vi "stateMachine_dualVStim_beta2.vi"() -> ()   [LabVIEW 2014]
uses:
  daq_channel_read_parameter.ctl
  <vilib>/Platform/TimedLoop/XDataNode/timing_clust.ctl
  <vilib>/Platform/TimedLoop/XDataNode/nitl_modes.ctl
  <vilib>/Platform/TimedLoop/XDataNode/wakeup.ctl
  <vilib>/dex/Stream Element Allocation Mode.ctl
  states_def.ctl
  UDP_Para_def.ctl
  <vilib>/DAQmx/write.llb/DAQmx Write (Digital 1D Bool NChan 1Samp 1Line).vi
  <vilib>/platform/TimedLoop/XDataNode/XDataNode.xnode
  <vilib>/Platform/TimedLoop/XDataNode/XDNodeRunTimeDep.lvlib
  <resource>/objmgr/ni.dex.rc
panel:
  out "rightcounter":i32
  out "leftcounter":i32
  out "beh type":string
  out "vs type":string
  out "Tab Control":enum32{"State Machine"}(tab)
  in  "No VS":bool
  in  "vsFilterPeriod_uS":i32=500 format="%#1.6f"
  in  "lickThreshold_V":fxp<+/-,16,5> format="%#.4g"
  in  "vsThreshold_V":fxp<+/-,16,5> format="%#.4g"
  in  "audioThreshold_V":fxp<+/-,16,5> format="%#.4g"
  in  "audioFilterPeriod_uS":i32=50000 format="%#1.6f"
  in  "audioOffState_V":fxp<+/-,16,5> format="%#.4g"
  out "rtFIFOsize":u32=50
  out "rtFIFOtimeout":u32
  out "rtFIFOdataPool":u32=50
  out "stateMachineCycle_uS":i64=500
  out "(Actual)":i64
  in  "delay_uS":u32
  out "IP_RT":string="192.168.137.2"
  in  "port_broadcast":u16=9091
  out "IP_host":string="192.168.137.1"
  out "port_host":u16=9090
  in  "Tab Control 2":enum32{"Data Transfer"}(tab)
  out "stream counter":u32
  out "Is Connected":bool
  out "Available Elements for Writing":i32
  out "stream writer buffer size":i32=500
  in  "rewardPeriod_uS":u32
  in  "waterOn_uS":u32
  in  "timeout_uS":u32=5000000
  in  "shockOn_uS":u32
  in  "Stop state":bool
  out "Initial data received":bool
  out "Tab Control 3":enum32{"Current status"}(tab)
  in  "toneReward":bool
  out "ABORT":bool
  out "trialStart":bool
  out "trialDone":bool
  out "Busy":bool
  out "stateLatched":bool
  out "curKey":u32=1
  out "curState":u32
  out "rtFIFOdataDim":i32
  in  "actuatorOn":bool
  in  "manualWaterRight":bool
  in  "manualWaterLeft":bool
  in  "lickReward":bool
  in  "allowPunish":bool
  in  "forceLRswitch":bool
  in  "allowCorrection":bool
  in  "allowAutoWater":bool
  out "error out":errorcluster
  in  "trialKey":i32[](array[numeric])
  in  "rwdrefPeriod_uS":u32
  out "FlagWaterLeft":bool
  in  "chanellParaCluster":T1={"audioOffState_V"=0.0, "audioFilterPeriod_uS"=50000, "audioThreshold_V"=0.0, "vsThreshold_V"=0.0, "vsFilterPeriod_uS"=0, "lickThreshold_V"=0.0} {"vsFilterPeriod_uS" format="%#1.6f"; "audioFilterPeriod_uS" format="%#1.6f"}
  out "leftWaterOnFlag":bool
  out "rightWaterOnFlag":bool
  out "contNoReward":i32
  out "rewardStatus":bool
  in  "timeVS_uS":u32=2000000
  in  "timeTravel_uS":i32=400000
  out "skipRewFlag":bool
types:
  T1 = typedef "daq_channel_read_parameter.ctl" = cluster{"audioOffState_V":fxp<+/-,16,5>, "audioFilterPeriod_uS":i32, "audioThreshold_V":fxp<+/-,16,5>, "vsThreshold_V":fxp<+/-,16,5>, "vsFilterPeriod_uS":i32, "lickThreshold_V":fxp<+/-,16,5>}
  T2 = typedef "XDNodeRunTimeDep.lvlib/timing_clust.ctl" = cluster{"Expected End [f-1]":u64, "Actual End [f-1]":u64, "Finished Late? [f-1]":bool, "Expected End [i-1]":u64, "Actual End [i-1]":u64, "Finished Late? [i-1]":bool, "Expected Start [i]":u64, "Actual Start [i]":u64, "Expected Start [f]":u64, "Actual Start [f]":u64, "Source Name":string, "Structure Name":string, "Period":i64, "Deadline":i64, "Offset":i64, "Start":i64, "Priority":i32, "Timeout":i32, "Mode":T3, "Wakeup Reason":T4, "Error":errorcluster, "Source Type":string, "Secondary Source Type":string, "Global End Time":u64, "Global Start Time":u64, "Frame Duration":u64, "Iteration Duration":u64, "Assigned CPU":i32, "I/O Scan Engine Mode":u32}
  T3 = typedef "XDNodeRunTimeDep.lvlib/nitl_modes.ctl" = enum32{"No Change", "Process missed periods, maintain original phase", "Discard missed periods, maintain original phase", "Process missed periods, ignore original phase", "Discard missed periods, ignore original phase"}
  T4 = typedef "XDNodeRunTimeDep.lvlib/wakeup.ctl" = enum32{"Normal", "Aborted", "Asynchronous wakeup", "Timing source error", "Timed loop error", "Timeout"}
  T5 = typedef "states_def.ctl" = enum16{"idle", "vs before", "vs", "vs after", "delay", "tone before", "tone", "tone after", "cycle end", "reward", "reward refractory", "punish", "punish refractory", "timeout", "exit", "manualwater"}
  T6 = typedef "Stream Element Allocation Mode.ctl" = u32
  T7 = typedef "UDP_Para_def.ctl" = enum16{"no", "start", "stop", "dly", "rwp", "rwf", "wdr", "shd", "tod", "lkr", "tlr", "alp", "msh", "mwl", "mwr", "alc", "lth", "vth", "ath", "aof", "afp", "vfp"}
  T8 = cluster{"leftLick":bool, "rightLick":bool, "visualStimuli2":bool, "tone":bool, "visualStimuli1":bool}
  T9 = cluster{"leftLick":dbl, "rightLick":dbl, "visualStimuli2":dbl, "tone":dbl, "visualStimuli1":dbl}
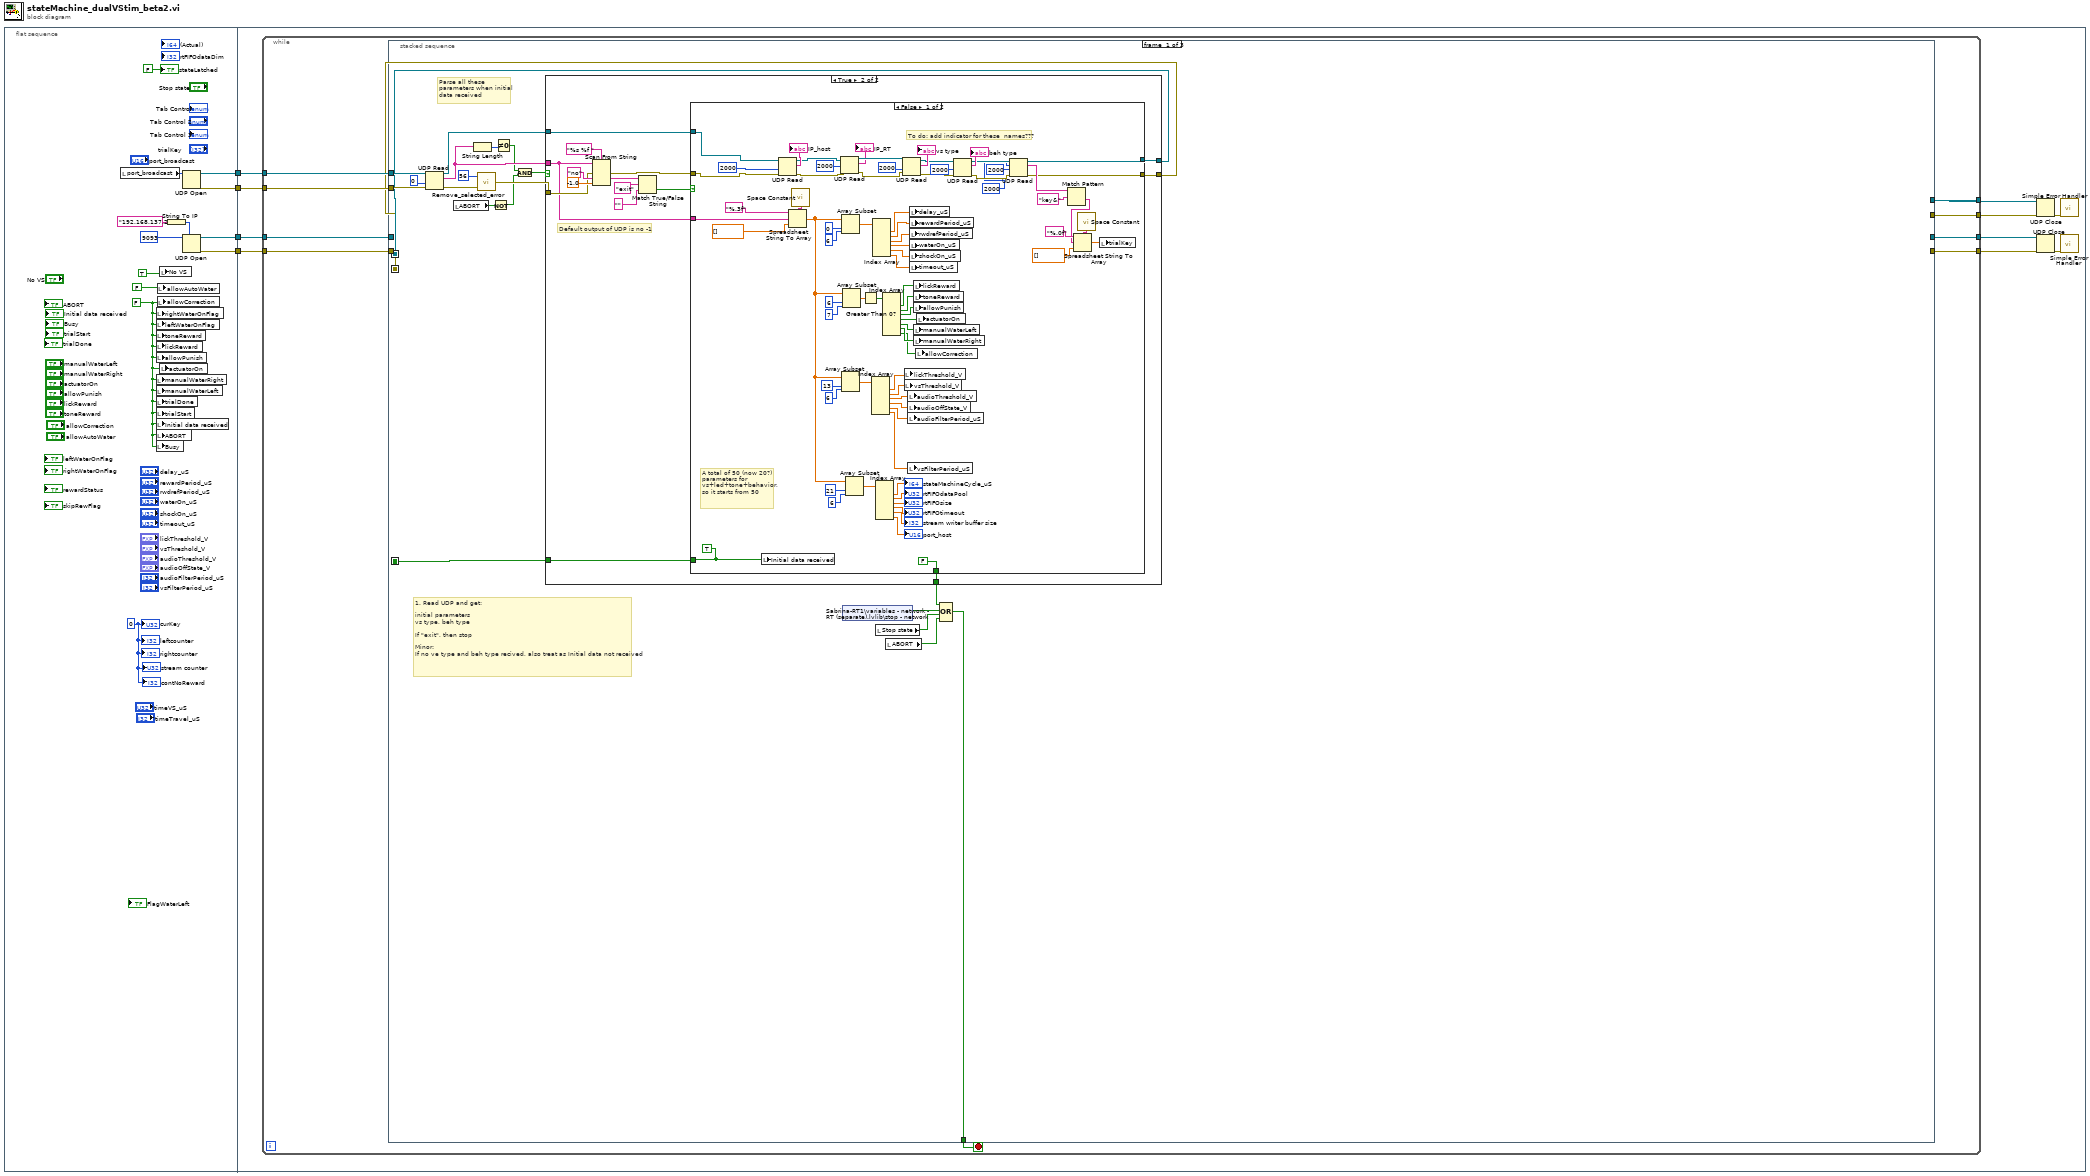
[diagram p0: block diagram]
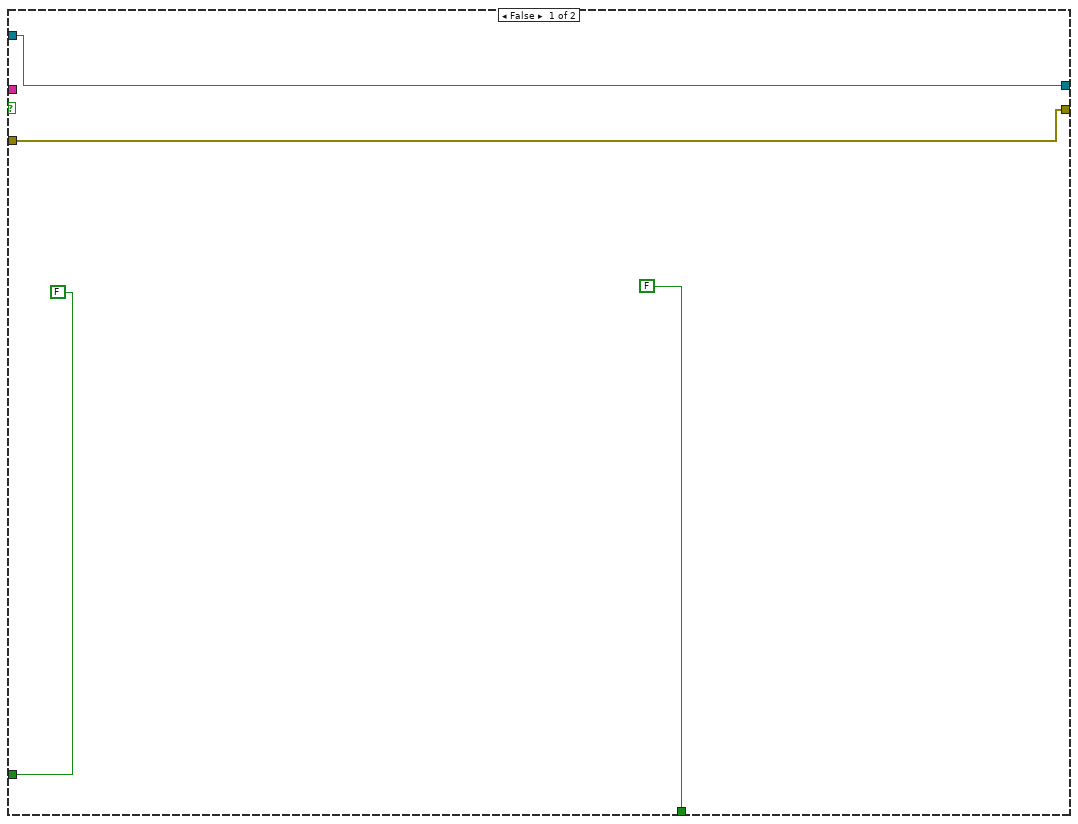
[diagram p2: hidden frame]
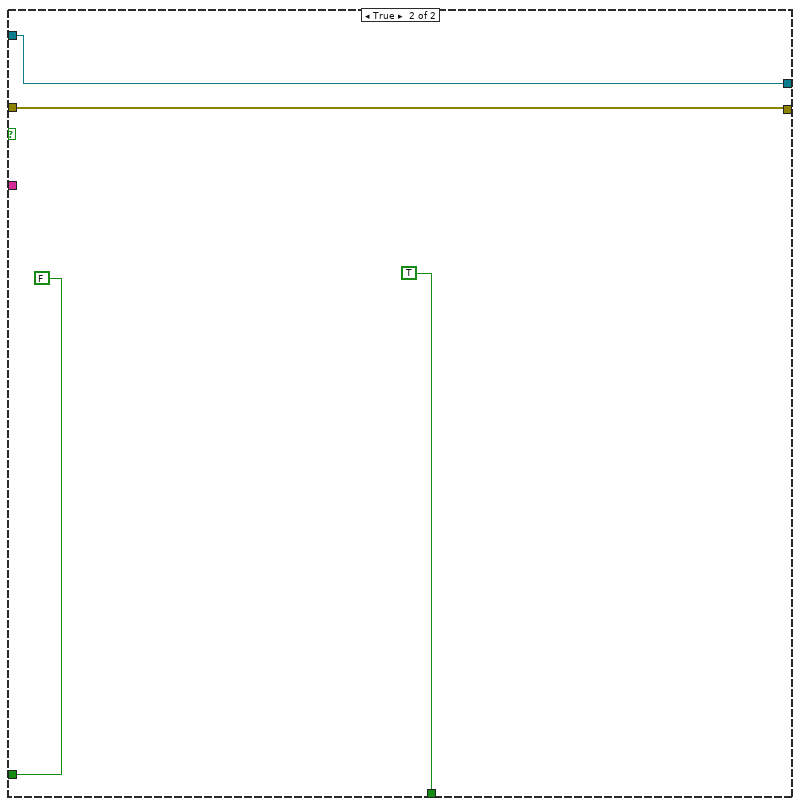
[diagram p3: hidden frame]
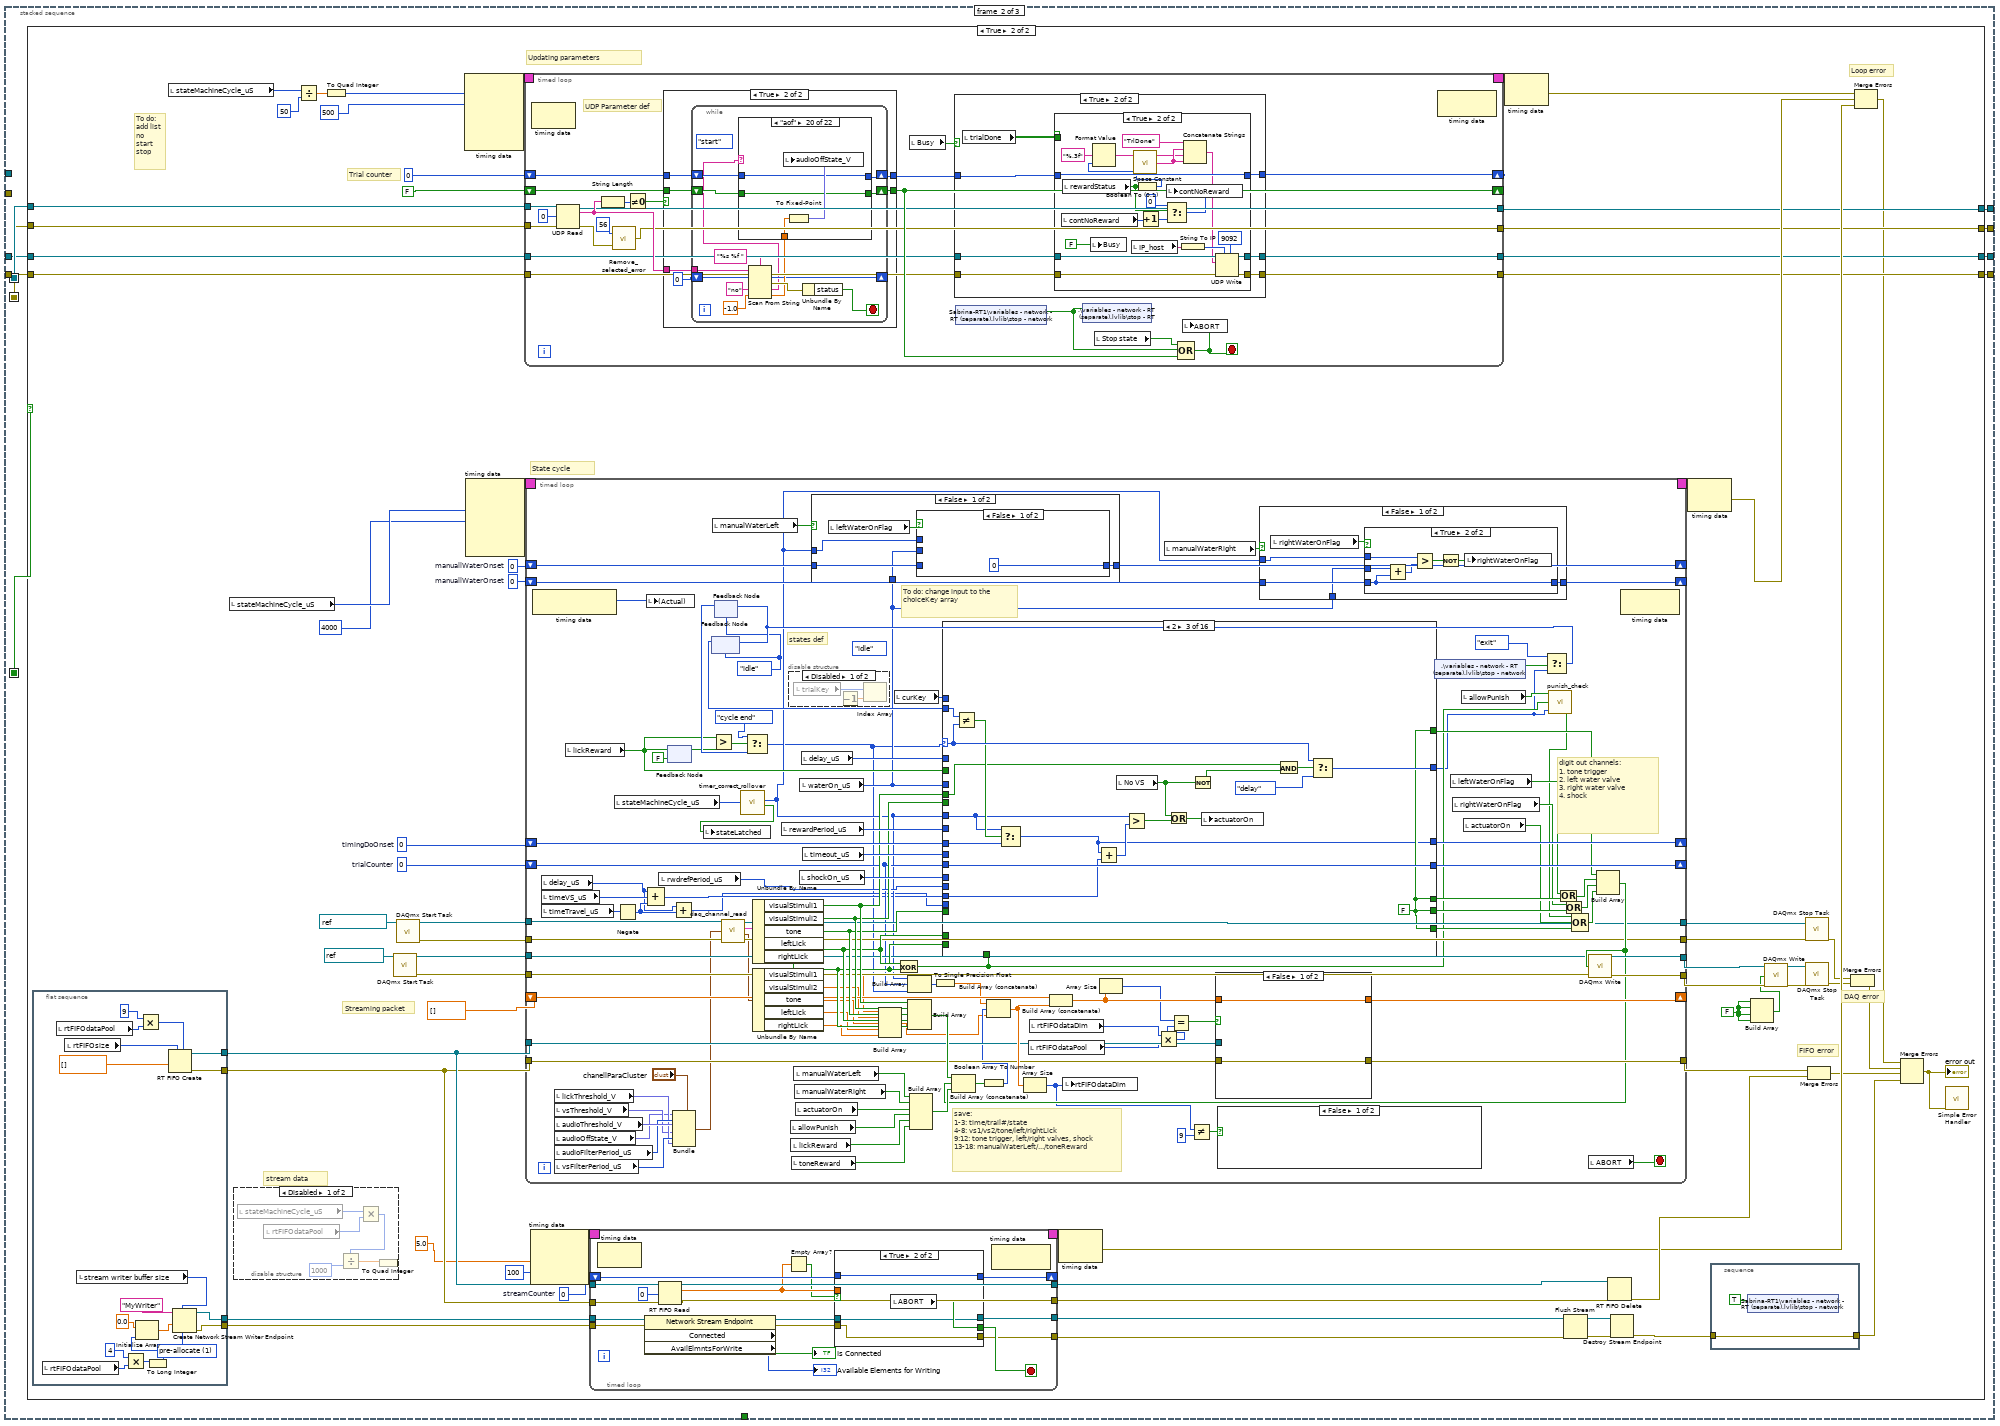
[diagram p4: hidden frame]
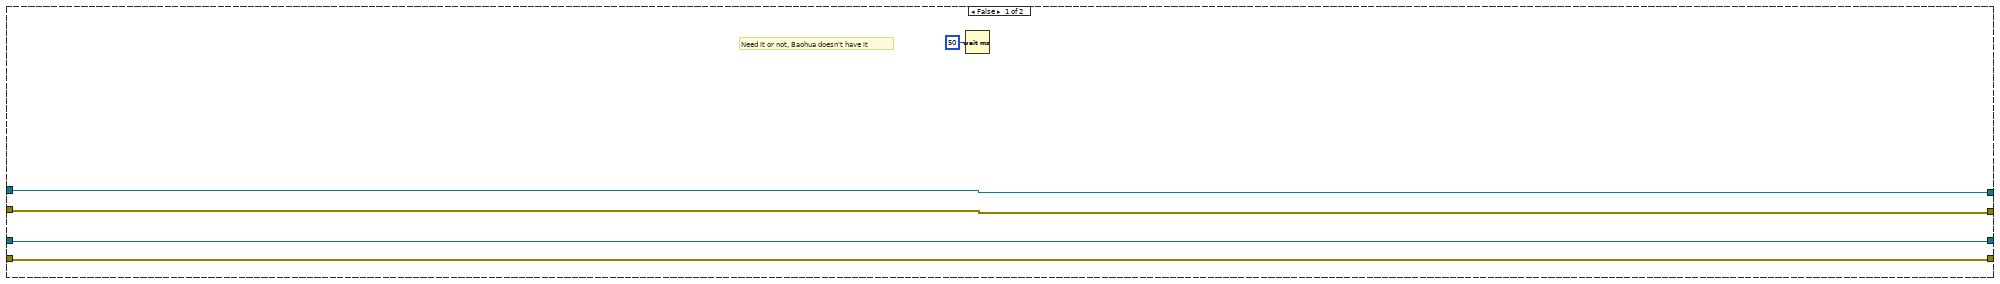
[diagram p5: hidden frame]
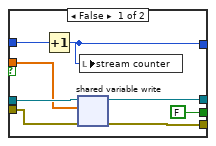
[diagram p7: hidden frame]
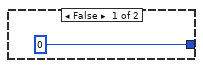
[diagram p9: hidden frame]
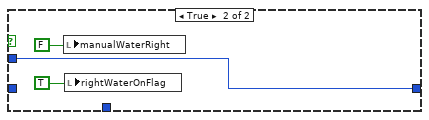
[diagram p10: hidden frame]
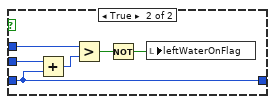
[diagram p11: hidden frame]
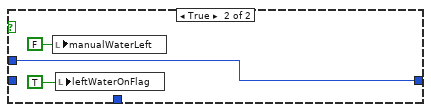
[diagram p12: hidden frame]
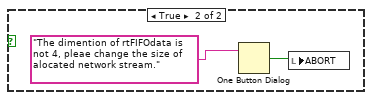
[diagram p13: hidden frame]
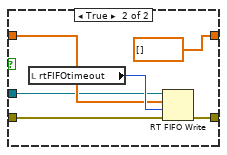
[diagram p14: hidden frame]
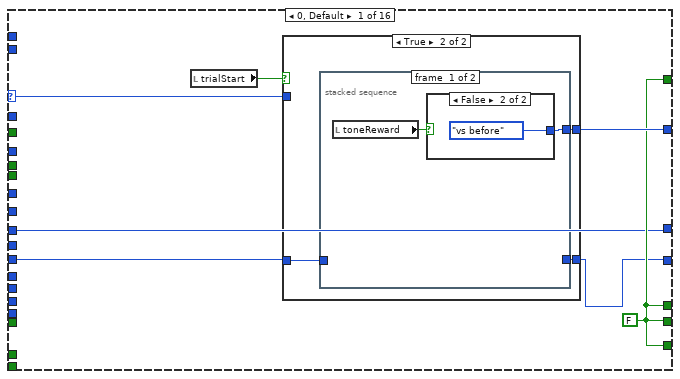
[diagram p15: hidden frame]
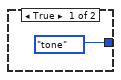
[diagram p17: hidden frame]
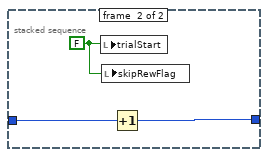
[diagram p18: hidden frame]
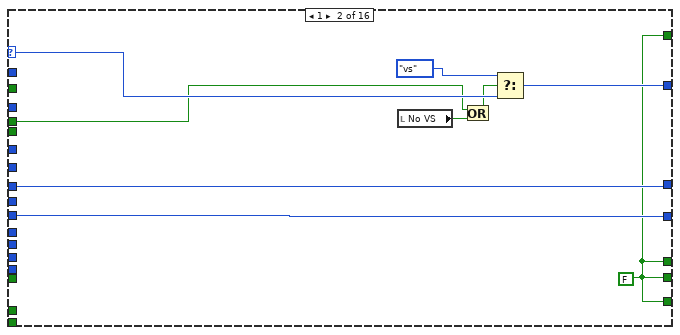
[diagram p19: hidden frame]
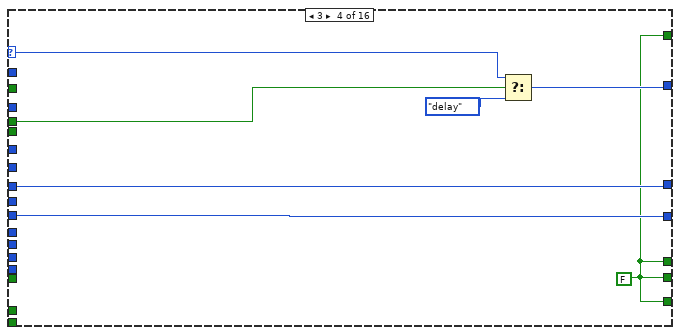
[diagram p20: hidden frame]
diagram:
  n1 = flat-sequence {
    tunnel: [w17] -> w4
    tunnel: [w16] -> w3
    tunnel: [w12] -> w2
    tunnel: [w11] -> w1
    tunnel: w4 -> [w27]
    tunnel: w3 -> [w26]
    tunnel: w2 -> [w22]
    tunnel: w1 -> [w21]
    frame #0 {
      w8 = FALSE
      w7 = 0
      n2 = local read "port_broadcast"() -> (w15:u16)
      n3 = local write "rightWaterOnFlag"(w8) -> ()
      n4 = local write "leftWaterOnFlag"(w8) -> ()
      n5 = local write "toneReward"(w8) -> ()
      n6 = local write "lickReward"(w8) -> ()
      n7 = local write "allowPunish"(w8) -> ()
      n8 = local write "manualWaterRight"(w8) -> ()
      n9 = local write "manualWaterLeft"(w8) -> ()
      n10 = local write "trialDone"(w8) -> ()
      n11 = local write "trialStart"(w8) -> ()
      n12 = local write "Initial data received"(w8) -> ()
      n13 = local write "ABORT"(w8) -> ()
      n14 = local write "Busy"(w8) -> ()
      n15 = local write "allowAutoWater"(FALSE) -> ()
      n16 = local write "allowCorrection"(w8) -> ()
      n17 = local write "No VS"(TRUE) -> ()
      n18 = local write "actuatorOn"(w8) -> ()
      n19 = String To IP(1:"192.168.137.2") -> (0:w9:u32)
      n20 = UDP Open(7:w9, 11:u16 9093) -> (port=w12:refnum<k16>, 0:w11:errorcluster)  [unwired: 3 in, 1 out]
      n21 = UDP Open(11:w15) -> (port=w17:refnum<k16>, 0:w16:errorcluster)  [unwired: 4 in, 1 out]
      "stateLatched" <- FALSE
      "curKey" <- w7
      "leftcounter" <- w7
      "rightcounter" <- w7
      "stream counter" <- w7
      "contNoReward" <- w7
    }
    frame #1 {
      n22 = while {
        tunnel: w27 -> [w36]
        tunnel: w26 -> [w35]
        tunnel: [w33] -> w24
        tunnel: [w32] -> w23
        tunnel: w22 -> [w31]
        tunnel: w21 -> [w30]
        tunnel: [w29] -> w20
        tunnel: [w28] -> w19
        stop <- w34 stop-if-true
        n23 = stacked-sequence {
          seq-local: [w46 _ _] -> [_ w163 _]
          seq-local: [w38 _ _] -> [_ w160 _]
          seq-local: [w37 _ _] -> [_ w159 _]
          tunnel: w36 -> [w57 _ _]
          tunnel: w35 -> [w56 _ _]
          tunnel: [w47 _ _] -> w34
          tunnel: [_ w162 _] -> w33
          tunnel: [_ w161 _] -> w32
          tunnel: w31 -> [_ w158 _]
          tunnel: w30 -> [_ w155 _]
          tunnel: [_ w157 _] -> w29
          tunnel: [_ w156 _] -> w28
          frame #0 {
            # "Parse all these \nparameters when initial\ndata received"
            # "1. Read UDP and get:\n\ninitial parameters\nvs type, beh type\n\nIf \"exit\", then stop\n\nMinor:\nIf no ve type and beh type recived, also treat as Initial data not received"
            n24 = UDP Read(connection ID=w57, timeout ms (25000)=0, 8:w56) -> (data out=w54:string, error out=w44:errorcluster, 3:w55:refnum<k16>)  [unwired: 1 in, 2 out]
            n25 = local read "ABORT"() -> (w42:bool)
            n26 = String Length(string=w54) -> (length=w53:i32)
            n27 = call "Remove_selected_error.vi"("error in (no error)"=w44, "errorCode"=56 ("timeout ms (25000)")) -> ("error out"=w45:errorcluster)
            n28 = Not(x=w42) -> (.not. x?=w39:bool)
            n29 = Not Equal To 0?(x=w53) -> (x != 0?=w40:bool)
            n30 = And(x=w40, y=w39) -> (x .and. y?=w41:bool)
            n31 = case shown="True" w41 {
              tunnel: w54 -> [_ w66]
              tunnel: w55 -> [w59 w67]
              tunnel: w45 -> [w58 w74]
              tunnel: [FALSE w65] -> w51
              tunnel: [FALSE w64] -> w46
              tunnel: [w59 w63] -> w38
              tunnel: [w58 w62] -> w37
              frame False {
              }
              frame True {
                # "Default output of UDP is no -1"
                n32 = Scan From String(format string="%s %f ", input string=w66, error in=w74, default 1="no" ("default value 1"), default 2=sgl -1.0 ("default value 1")) -> (error out=w68:errorcluster, output 1=w73:string)  [unwired: 2 in, 2 out]
                n33 = Match True/False String(2:"" ("false string"), 3:"exit" ("true string"), 4:w73) -> (0:w69:bool)  [unwired: 1 out]
                n34 = case shown="False" w69 {
                  tunnel: w68 -> [w112 w152]
                  tunnel: w67 -> [w113 w151]
                  tunnel: w66 -> [w144 _]
                  tunnel: [FALSE TRUE] -> w65
                  tunnel: [w142 FALSE] -> w64
                  tunnel: [w79 w151] -> w63
                  tunnel: [w78 w152] -> w62
                  frame False {
                    w142 = TRUE
                    # "A total of 50 (now 20?) parameters for vs+led+tone+behavior, so it starts from 50"
                    # "To do: add indicator for these  names???"
                    n35 = local write "Initial data received"(w142) -> ()
                    n36 = UDP Read(connection ID=w113, timeout ms (25000)=2000, 8:w112) -> (data out=→"IP_host":string, error out=w111:errorcluster, 3:w109:refnum<k16>)  [unwired: 1 in, 2 out]
                    n37 = call <vilib>:"Space Constant.vi"() -> ("String"=w149:string)
                    n38 = Spreadsheet String To Array(delimiter (Tab)=w149, format string="%.3f", spreadsheet string=w144, array type (2D Dbl)=sgl[] []) -> (array=w120:sgl[])
                    n39 = UDP Read(connection ID=w109, timeout ms (25000)=2000, 8:w111) -> (data out=→"IP_RT":string, error out=w110:errorcluster, 3:w108:refnum<k16>)  [unwired: 1 in, 2 out]
                    n40 = Array Subset(array=w120, index=0 ("timeout ms (25000)"), length=6 ("timeout ms (25000)")) -> (w138:sgl[])
                    n41 = Array Subset(array=w120, index=13 ("timeout ms (25000)"), length=6 ("timeout ms (25000)")) -> (w134:sgl[])
                    n42 = Array Subset(array=w120, index=6 ("timeout ms (25000)"), length=7 ("timeout ms (25000)")) -> (w131:sgl[])
                    n43 = Array Subset(array=w120, index=21 ("timeout ms (25000)"), length=6 ("timeout ms (25000)")) -> (w121:sgl[])
                    n44 = Greater Than 0?(x=w131) -> (x > 0?=w130:bool[])
                    n45 = Index Array(array=w134) -> (element #1=w96:sgl, element #2=w95:sgl, element #3=w94:sgl, element #4=w93:sgl, element #5=w92:sgl, element #6=w91:sgl)  [unwired: 6 in]
                    n46 = Index Array(array=w138) -> (element #1=w102:sgl, element #2=w101:sgl, element #3=w100:sgl, element #4=w99:sgl, element #5=w98:sgl, element #6=w97:sgl)  [unwired: 6 in]
                    n47 = Index Array(array=w121) -> (element #1=→"stateMachineCycle_uS":sgl, element #2=→"rtFIFOdataPool":sgl, element #3=→"rtFIFOsize":sgl, element #4=→"rtFIFOtimeout":sgl, element #5=→"stream writer buffer size":sgl, element #6=→"port_host":sgl)  [unwired: 6 in]
                    n48 = Index Array(array=w130) -> (element #1=w129:bool, element #2=w128:bool, element #3=w127:bool, element #4=w126:bool, element #5=w125:bool, element #6=w124:bool, element #7=w77:bool)  [unwired: 7 in]
                    n49 = UDP Read(connection ID=w108, timeout ms (25000)=2000, 8:w110) -> (data out=→"vs type":string, error out=w141:errorcluster, 3:w140:refnum<k16>)  [unwired: 1 in, 2 out]
                    n50 = local write "lickThreshold_V"(w96) -> ()
                    n51 = local write "vsThreshold_V"(w95) -> ()
                    n52 = local write "audioThreshold_V"(w94) -> ()
                    n53 = local write "audioOffState_V"(w93) -> ()
                    n54 = local write "audioFilterPeriod_uS"(w92) -> ()
                    n55 = local write "vsFilterPeriod_uS"(w91) -> ()
                    n56 = local write "delay_uS"(w102) -> ()
                    n57 = local write "rewardPeriod_uS"(w101) -> ()
                    n58 = local write "rwdrefPeriod_uS"(w100) -> ()
                    n59 = local write "waterOn_uS"(w99) -> ()
                    n60 = local write "shockOn_uS"(w98) -> ()
                    n61 = local write "timeout_uS"(w97) -> ()
                    n62 = local write "lickReward"(w129) -> ()
                    n63 = local write "toneReward"(w128) -> ()
                    n64 = local write "allowPunish"(w127) -> ()
                    n65 = local write "manualWaterLeft"(w125) -> ()
                    n66 = local write "manualWaterRight"(w124) -> ()
                    n67 = local write "allowCorrection"(w77) -> ()
                    n68 = local write "actuatorOn"(w126) -> ()
                    n69 = UDP Read(connection ID=w140, timeout ms (25000)=2000, 8:w141) -> (data out=→"beh type":string, error out=w88:errorcluster, 3:w89:refnum<k16>)  [unwired: 1 in, 2 out]
                    n70 = UDP Read(connection ID=w89, max size (548)=2000 ("timeout ms (25000)"), timeout ms (25000)=2000, 8:w88) -> (data out=w83:string, error out=w78:errorcluster, 3:w79:refnum<k16>)  [unwired: 2 out]
                    n71 = Match Pattern(string=w83, regular expression="key&") -> (after substring=w81:string)  [unwired: 1 in, 3 out]
                    n72 = call <vilib>:"Space Constant.vi"() -> ("String"=w86:string)
                    n73 = Spreadsheet String To Array(delimiter (Tab)=w86, format string="%.0f", spreadsheet string=w81, array type (2D Dbl)=dbl[] []) -> (array=w84:dbl[])
                    n74 = local write "trialKey"(w84) -> ()
                  }
                  frame True {
                  }
                }
              }
            }
            n75 = shared-variable "Sabrina-RT1\\variables - network - RT (separate).lvlib\\stop - network"() -> (w50:bool)  [unwired: 1 in, 1 out]
            n76 = local read "Stop state"() -> (w49:bool)
            n77 = local read "ABORT"() -> (w48:bool)
            n78 = Compound Arithmetic op=OR(w51, w50, w49, w48) -> (w47:bool)
          }
          frame #1 {
            n79 = case shown="True" w163 {
              tunnel: w160 -> [w167 w213]
              tunnel: w159 -> [w166 w212]
              tunnel: [w167 w185] -> w162
              tunnel: [w166 w186] -> w161
              tunnel: w158 -> [w165 w190]
              tunnel: w155 -> [w164 w189]
              tunnel: [w164 w188] -> w157
              tunnel: [w165 w187] -> w156
              frame False {
                # "Need it or not, Baohua doesn't have it"
                n80 = Wait (ms)(milliseconds to wait=u32 50) -> ()  [unwired: 1 out]
              }
              frame True {
                w169 = 0  # manuallWaterOnset
                w170 = 0  # manuallWaterOnset
                w196 = FALSE
                w225 = 0  # streamCounter
                w228 = 0  # timingDoOnset
                w227 = 0  # trialCounter
                # "Streaming packet"
                # "Trial counter"
                # "Loop error"
                # "DAQ error"
                # "FIFO error"
                # "Updating parameters"
                # "State cycle"
                # "To do:\nadd list\nno\nstart\nstop"
                # "stream data"
                n81 = flat-sequence {
                  tunnel: [w255] -> w230
                  tunnel: [w254] -> w229
                  tunnel: [w253] -> w216
                  tunnel: [w252] -> w215
                  frame #0 {
                    w259 = T6 1 items=["allocate as needed", "pre-allocate"] ("element allocation mode")
                    n82 = local read "rtFIFOdataPool"() -> (w250:u32)
                    n83 = local read "rtFIFOdataPool"() -> (w247:u32)
                    n84 = local read "rtFIFOsize"() -> (w261:u32)
                    n85 = local read "stream writer buffer size"() -> (w251:i32)
                    n86 = Multiply(x=u32 4, y=w250) -> (x*y=w245:u32)
                    n87 = Multiply(x=9, y=w247) -> (x*y=w246:u32)
                    n88 = To Long Integer(number=w245) -> (32bit integer=w244:i32)
                    n89 = Initialize Array(sgl 0.0, w244) -> (w258:sgl[])
                    n90 = RT FIFO Create(1:sgl[] [], 4:w261, 6:w246) -> (8:w253:refnum<k33>, 11:w252:errorcluster)  [unwired: 5 in, 1 out]
                    n91 = Create Network Stream Writer Endpoint(6:w259, 7:w251, 9:w258, 11:"MyWriter" ("writer name")) -> (0:w255:errorcluster, 3:w254:refnum<k21>)  [unwired: 3 in]
                  }
                }
                n92 = local read "stateMachineCycle_uS"() -> (w214:i64)
                n93 = local read "stateMachineCycle_uS"() -> (w224:i64)
                n94 = disable-structure shown="Disabled" {
                  frame Disabled {
                    n95 = local read "stateMachineCycle_uS"() -> (w239:i64)
                    n96 = local read "rtFIFOdataPool"() -> (w238:u32)
                    n97 = Multiply(x=w239, y=w238) -> (x*y=w240:i64)
                    n98 = Divide(x=w240, y=i64 1000) -> (x/y=w237:dbl)
                    n99 = To Quad Integer(1:w237) -> ()  [unwired: 1 out]
                  }
                  frame Enabled {
                  }
                }
                n100 = Divide(x=w214, y=i64 50) -> (x/y=w220:dbl)
                n101 = To Quad Integer(1:w220) -> (0:w219:i64)
                n102 = call <vilib>:"DAQmx Start Task.vi"("task/channels in"=refnum<k21> "digitWrite" ("digitWrite")) -> ("task out"=w182:refnum<k21>, "error out"=w181:errorcluster)  [unwired: 13 in]
                n103 = call <vilib>:"DAQmx Start Task.vi"("task/channels in"=refnum<k21> "analogRead" ("DAQmx Task Name")) -> ("task out"=w172:refnum<k21>, "error out"=w171:errorcluster)  [unwired: 13 in]
                n104 = node-c288(w219, 500 ("Priority")) -> (w236:T2)  [unwired: 3 in]
                n105 = node-c288(w224, 4000 ("Priority")) -> (w234:T2)  [unwired: 3 in]
                n106 = timed-loop {
                  timing: w236 -> [_]
                  timing-out: [_] -> w235
                  shift-right: [w768] -> _
                  shift-left: 0 ("timeout ms (25000)") -> [w770]
                  shift-right: [w764] -> _
                  shift-left: FALSE -> [w767]
                  tunnel: [w761] -> w187
                  tunnel: [w760] -> w188
                  tunnel: w213 -> [w759]
                  tunnel: w212 -> [w758]
                  tunnel: w190 -> [w752]
                  tunnel: w189 -> [w755]
                  tunnel: [w754] -> w186
                  tunnel: [w753] -> w185
                  stop <- w766 stop-if-true
                  # "UDP Parameter def"
                  n107 = node-c288() -> ()  [unwired: 1 in, 1 out]
                  n108 = UDP Read(connection ID=w759, timeout ms (25000)=0, 8:w758) -> (data out=w771:string, error out=w757:errorcluster, 3:w753:refnum<k16>)  [unwired: 1 in, 2 out]
                  n109 = String Length(string=w771) -> (length=w773:i32)
                  n110 = call "Remove_selected_error.vi"("error in (no error)"=w757, "errorCode"=56 ("timeout ms (25000)")) -> ("error out"=w754:errorcluster)
                  n111 = Not Equal To 0?(x=w773) -> (x != 0?=w772:bool)
                  n112 = case shown="True" w772 {
                    tunnel: w771 -> [_ w815]
                    tunnel: w770 -> [w809 w814]
                    tunnel: [w809 w813] -> w769
                    tunnel: w767 -> [w808 w812]
                    tunnel: [w808 w811] -> w764
                    frame False {
                    }
                    frame True {
                      n113 = while {
                        tunnel: w815 -> [w829]
                        shift-right: [w817] -> _
                        shift-left: 0 ("timeout ms (25000)") -> [w818]
                        shift-right: [w822] -> w813
                        shift-left: w814 -> [w823]
                        shift-right: [w820] -> w811
                        shift-left: w812 -> [w821]
                        stop <- w824 stop-if-true
                        (unwired) UDP_Para_def."start"
                        n114 = Scan From String(format string="%s %f ", input string=w829, initial scan location=w818, default 1="no" ("default value 1"), default 2=-1.0 ("default value 2")) -> (offset past scan=w817:u32, error out=w825:errorcluster, output 1=w816:string, output 2=w819:dbl)  [unwired: 1 in, 1 out]
                        n115 = case shown="\"aof\"" w816 {
                          tunnel: [w831 w833 w842 w844 w849 w854 w859 w864 w869 w874 w878 w882 w886 w890 w894 w899 w902 w906 w910 w914 w918 w923] -> w822
                          tunnel: w823 -> [w831 w834 w842 w844 w849 w854 w859 w864 w869 w874 w878 w882 w886 w890 w894 w899 w902 w906 w910 w914 w918 w923]
                          tunnel: [w830 w838 w839 w843 w848 w853 w858 w863 w868 w873 w877 w881 w885 w889 w893 w898 w901 w905 w909 w913 w917 w922] -> w820
                          tunnel: w821 -> [w830 w838 w840 w843 w848 w853 w858 w863 w868 w873 w877 w881 w885 w889 w893 w898 w901 w905 w909 w913 w917 w922]
                          tunnel: w819 -> [_ w835 _ w846 w851 w856 w861 w866 w871 w876 w880 w884 w888 w892 w896 w900 w904 w908 w912 w916 w920 w925]
                          frame "no", Default {
                          }
                          frame "start" {
                            w837 = TRUE
                            n116 = Increment(x=w834) -> (x+1=w833:i32)
                            n117 = local write "rewardStatus"(FALSE) -> ()
                            n118 = local write "trialDone"(FALSE) -> ()
                            n119 = local write "Busy"(w837) -> ()
                            n120 = local write "trialStart"(w837) -> ()
                            n121 = local write "curKey"(w835) -> ()
                          }
                          frame "stop" {
                            n122 = Or(x=w840, y=TRUE) -> (x .or. y?=w839:bool)
                          }
                          frame "dly" {
                            n123 = Multiply(x=1.0, y=w846) -> (x*y=w845:dbl)
                            n124 = local write "delay_uS"(w845) -> ()
                          }
                          frame "rwp" {
                            n125 = Multiply(x=1.0, y=w851) -> (x*y=w850:dbl)
                            n126 = local write "rewardPeriod_uS"(w850) -> ()
                          }
                          frame "rwf" {
                            n127 = Multiply(x=1.0, y=w856) -> (x*y=w855:dbl)
                            n128 = local write "rwdrefPeriod_uS"(w855) -> ()
                          }
                          frame "wdr" {
                            n129 = Multiply(x=1.0, y=w861) -> (x*y=w860:dbl)
                            n130 = local write "waterOn_uS"(w860) -> ()
                          }
                          frame "shd" {
                            n131 = Multiply(x=1.0, y=w866) -> (x*y=w865:dbl)
                            n132 = local write "shockOn_uS"(w865) -> ()
                          }
                          frame "tod" {
                            n133 = Multiply(x=1.0, y=w871) -> (x*y=w870:dbl)
                            n134 = local write "timeout_uS"(w870) -> ()
                          }
                          frame "lkr" {
                            n135 = Greater Than 0?(x=w876) -> (x > 0?=w875:bool)
                            n136 = local write "lickReward"(w875) -> ()
                          }
                          frame "tlr" {
                            n137 = Greater Than 0?(x=w880) -> (x > 0?=w879:bool)
                            n138 = local write "toneReward"(w879) -> ()
                          }
                          frame "alp" {
                            n139 = Greater Than 0?(x=w884) -> (x > 0?=w883:bool)
                            n140 = local write "allowPunish"(w883) -> ()
                          }
                          frame "msh" {
                            n141 = Greater Than 0?(x=w888) -> (x > 0?=w887:bool)
                            n142 = local write "actuatorOn"(w887) -> ()
                          }
                          frame "mwl" {
                            n143 = Greater Than 0?(x=w892) -> (x > 0?=w891:bool)
                            n144 = local write "manualWaterLeft"(w891) -> ()
                          }
                          frame "mwr" {
                            n145 = Greater Than 0?(x=w896) -> (x > 0?=w895:bool)
                            n146 = local write "manualWaterRight"(w895) -> ()
                          }
                          frame "alc" {
                            n147 = Greater Than 0?(x=w900) -> (x > 0?=w897:bool)
                            n148 = local write "allowCorrection"(w897) -> ()
                          }
                          frame "lth" {
                            n149 = To Fixed-Point(number=w904) -> (fixed-point=w903:fxp<+/-,32,16>)  [unwired: 1 in]
                            n150 = local write "lickThreshold_V"(w903) -> ()
                          }
                          frame "vth" {
                            n151 = To Fixed-Point(number=w908) -> (fixed-point=w907:fxp<+/-,32,16>)  [unwired: 1 in]
                            n152 = local write "vsThreshold_V"(w907) -> ()
                          }
                          frame "ath" {
                            n153 = To Fixed-Point(number=w912) -> (fixed-point=w911:fxp<+/-,32,16>)  [unwired: 1 in]
                            n154 = local write "audioThreshold_V"(w911) -> ()
                          }
                          frame "aof" {
                            n155 = To Fixed-Point(number=w916) -> (fixed-point=w915:fxp<+/-,32,16>)  [unwired: 1 in]
                            n156 = local write "audioOffState_V"(w915) -> ()
                          }
                          frame "afp" {
                            n157 = Multiply(x=1.0, y=w920) -> (x*y=w919:dbl)
                            n158 = local write "audioFilterPeriod_uS"(w919) -> ()
                          }
                          frame "vfp" {
                            n159 = Multiply(x=1.0, y=w925) -> (x*y=w924:dbl)
                            n160 = local write "vsFilterPeriod_uS"(w924) -> ()
                          }
                        }
                        n161 = Unbundle By Name(w825) -> ("status"=w824:bool)
                      }
                    }
                  }
                  n162 = local read "Busy"() -> (w765:bool)
                  n163 = case shown="True" w765 {
                    tunnel: w769 -> [w777 w784]
                    tunnel: [w777 w778] -> w768
                    tunnel: w752 -> [w776 w783]
                    tunnel: [w776 w782] -> w761
                    tunnel: [w775 w781] -> w760
                    tunnel: w755 -> [w775 w780]
                    frame False {
                    }
                    frame True {
                      n164 = local read "trialDone"() -> (w779:bool)
                      n165 = case shown="True" w779 {
                        tunnel: w784 -> [w787 w802]
                        tunnel: [w787 w802] -> w778
                        tunnel: w783 -> [w786 w801]
                        tunnel: [w786 w800] -> w782
                        tunnel: [w785 w799] -> w781
                        tunnel: w779 -> [_ _]
                        tunnel: w780 -> [w785 w796]
                        frame False {
                        }
                        frame True {
                          n166 = local read "contNoReward"() -> (w790:i32)
                          n167 = local read "rewardStatus"() -> (w792:bool)
                          n168 = local write "Busy"(FALSE) -> ()
                          n169 = local read "IP_host"() -> (w797:string)
                          n170 = call <vilib>:"Space Constant.vi"() -> ("String"=w806:string)
                          n171 = Boolean To (0,1)(Boolean=w792) -> (0, 1=w793:i16)
                          n172 = Format Value(format string="%.3f", value (0)=w793) -> (output string=w804:string)  [unwired: 1 in]
                          n173 = Increment(x=w790) -> (x+1=w789:i32)
                          n174 = Select(t=0 ("timeout ms (25000)"), s=w792, f=w789) -> (s? t:f=w788:i32)
                          n175 = local write "contNoReward"(w788) -> ()
                          n176 = String To IP(1:w797) -> (0:w803:u32)
                          n177 = Concatenate Strings("TrlDone" ("data in"), w806, w804, w806) -> (w795:string)
                          n178 = UDP Write(address=w803, port or service name=u16 9092, connection ID=w801, data in=w795, 8:w796) -> (error out=w799:errorcluster, 3:w800:refnum<k16>)  [unwired: 1 in]
                        }
                      }
                    }
                  }
                  n179 = shared-variable "Sabrina-RT1\\variables - network - RT (separate).lvlib\\stop - network"() -> (w763:bool)  [unwired: 1 in, 1 out]
                  n180 = shared-variable ".\\variables - network - RT (separate).lvlib\\stop - RT"(w763) -> ()  [unwired: 1 in, 1 out]
                  n181 = local read "Stop state"() -> (w762:bool)
                  n182 = Compound Arithmetic op=OR(w762, w763, w764) -> (w766:bool)
                  n183 = local write "ABORT"(w766) -> ()
                  n184 = node-c288() -> ()  [unwired: 1 in, 1 out]
                }
                n185 = timed-loop {
                  timing: w234 -> [_]
                  timing-out: [_] -> w233
                  shift-right: [w393] -> _
                  shift-left: w227 -> [w331]
                  tunnel: [w404] -> w203
                  tunnel: [w403] -> w202
                  shift-right: [w401] -> _
                  shift-left: w228 -> [w402]
                  tunnel: w172 -> [w395]
                  tunnel: w171 -> [w361]
                  tunnel: [w333] -> w177
                  shift-right: [w386] -> _
                  shift-left: sgl[] [] ("array type (2D Dbl)") -> [w387]
                  tunnel: [w383] -> w193
                  tunnel: w216 -> [w360]
                  tunnel: w215 -> [w359]
                  tunnel: w182 -> [w349]
                  tunnel: w181 -> [w348]
                  tunnel: [w343] -> w178
                  shift-right: [w321] -> _
                  shift-left: w170 -> [w322]
                  shift-right: [w317] -> _
                  shift-left: w169 -> [w318]
                  stop <- w344 stop-if-true
                  w353 = states_def."idle"
                  (unwired) states_def."idle"
                  # "states def"
                  # "save: \n1-3: time/trail#/state\n4-8: vs1/vs2/tone/left/rightLick\n9:12: tone trigger, left/right valves, shock\n13-18: manualWaterLeft/.../toneReward"
                  # "digit out channels:\n1. tone trigger\n2. left water valve\n3. right water valve\n4. shock"
                  # "To do: change input to the choiceKey array"
                  n186 = node-c288() -> (w356:i64)  [unwired: 1 in]
                  n187 = local read "delay_uS"() -> (w302:u32)
                  n188 = local read "timeVS_uS"() -> (w306:u32)
                  n189 = local read "timeTravel_uS"() -> (w305:i32)
                  n190 = local read "lickThreshold_V"() -> (w337:fxp<+/-,16,5>)
                  n191 = local read "vsThreshold_V"() -> (w336:fxp<+/-,16,5>)
                  n192 = local read "audioThreshold_V"() -> (w342:fxp<+/-,16,5>)
                  n193 = local read "audioOffState_V"() -> (w335:fxp<+/-,16,5>)
                  n194 = local read "audioFilterPeriod_uS"() -> (w338:i32)
                  n195 = local read "vsFilterPeriod_uS"() -> (w339:i32)
                  n196 = local read "lickReward"() -> (w362:bool)
                  n197 = local read "stateMachineCycle_uS"() -> (w357:i64)
                  n198 = Negate(x=w305) -> (-x=w303:i32)
                  n199 = local write "(Actual)"(w356) -> ()
                  n200 = Compound Arithmetic op=ADD(w302, w306, w303) -> (w304:u32)
                  n201 = local read "rwdrefPeriod_uS"() -> (w350:u32)
                  n202 = feedback #1(FALSE ("lick-reward")) -> (w407:bool)
                  n203 = feedback-in #1(w362) -> ()
                  n204 = Add(x=w302, y=w303) -> (x+y=w301:u32)
                  n205 = Bundle(cluster="chanellParaCluster", "audioOffState_V"=w335, "audioFilterPeriod_uS"=w338, "audioThreshold_V"=w342, "vsThreshold_V"=w336, "vsFilterPeriod_uS"=w339, "lickThreshold_V"=w337) -> (w341:T1)
                  n206 = feedback #2(w353) -> (w405:u32)
                  n207 = Greater?(x=w362, y=w407) -> (0:w408:bool)
                  n208 = local read "manualWaterLeft"() -> (w323:bool)
                  n209 = feedback #3(w353) -> (w409:u32)
                  n210 = call "daq_channel_read.vi"("DAQmxTaskIn"=w395, "chanellParaCluster"=w341, "error in (no error)"=w361) -> ("DAQmxTaskOut"=w343:refnum<k21>, "channelOutCluster"=w334:T8, "channelOutCluster_rawData"=w332:T9, "error out"=w333:errorcluster)
                  n211 = call "timer_correct_rollover.vi"("Loop Rate(uSec)"=w357) -> ("Late? (Latched)"=w396:bool, "Tick Count(uSec)"=w316:u64)  [unwired: 8 in, 1 out]
                  n212 = local write "stateLatched"(w396) -> ()
                  n213 = Select(t=states_def."cycle end", s=w408, f=w409) -> (s? t:f=w300:u32)
                  n214 = Unbundle By Name(w334) -> ("visualStimuli1"=w392:bool, "visualStimuli2"=w391:bool, "tone"=w390:bool, "leftLick"=w389:bool, "rightLick"=w388:bool)
                  n215 = Unbundle By Name(w332) -> ("visualStimuli1"=w325:dbl, "visualStimuli2"=w330:dbl, "tone"=w329:dbl, "leftLick"=w328:dbl, "rightLick"=w327:dbl)
                  n216 = local read "rewardPeriod_uS"() -> (w399:u32)
                  n217 = disable-structure shown="Disabled" {
                    frame Disabled {
                      n218 = local read "trialKey"() -> (w412:i32[])
                      n219 = Decrement() -> (x-1=w411:dbl)  [unwired: 1 in]
                      n220 = Index Array(array=w412, index=w411) -> ()  [unwired: 1 out]
                    }
                    frame Enabled {
                    }
                  }
                  n221 = local read "allowPunish"() -> (w371:bool)
                  n222 = local read "lickReward"() -> (w372:bool)
                  n223 = local read "toneReward"() -> (w351:bool)
                  n224 = local read "manualWaterLeft"() -> (w369:bool)
                  n225 = local read "manualWaterRight"() -> (w368:bool)
                  n226 = local read "actuatorOn"() -> (w370:bool)
                  n227 = local read "shockOn_uS"() -> (w394:u32)
                  n228 = local read "waterOn_uS"() -> (w315:u32)
                  n229 = local read "delay_uS"() -> (w352:u32)
                  n230 = local read "timeout_uS"() -> (w398:u32)
                  n231 = case shown="False" w323 {
                    tunnel: w322 -> [w431 _]
                    tunnel: [w430 w442] -> w321
                    tunnel: w316 -> [w429 w442]
                    tunnel: w315 -> [w428 _]
                    frame False {
                      n232 = local read "leftWaterOnFlag"() -> (w432:bool)
                      n233 = case shown="False" w432 {
                        tunnel: w431 -> [_ w437]
                        tunnel: [0 w437] -> w430
                        tunnel: w429 -> [_ w439]
                        tunnel: w428 -> [_ w438]
                        frame False {
                        }
                        frame True {
                          n234 = Add(x=w438, y=w437) -> (x+y=w436:u64)
                          n235 = Greater?(x=w439, y=w436) -> (0:w435:bool)
                          n236 = Not(x=w435) -> (.not. x?=w434:bool)
                          n237 = local write "leftWaterOnFlag"(w434) -> ()
                        }
                      }
                    }
                    frame True {
                      n238 = local write "manualWaterLeft"(FALSE) -> ()
                      n239 = local write "leftWaterOnFlag"(TRUE) -> ()
                    }
                  }
                  n240 = Build Array(w325, w330, w329, w328, w327) -> (w324:dbl[])
                  n241 = local read "curKey"() -> (w313:u32)
                  n242 = Exclusive Or(1:w388, 2:w389) -> (0:w309:bool)
                  n243 = Build Array(w316, w331, w300) -> (w366:u64[])
                  n244 = Build Array(w392, w391, w390, w389, w388) -> (w376:bool[])
                  n245 = Build Array(w369, w368, w370, w371, w372, w351) -> (w375:bool[])
                  n246 = To Single Precision Float(number=w366) -> (single precision float=w367:sgl[])
                  n247 = case shown="2" w300 {
                    selector: w300 -> [w456 w479 w493 w505 w522 w538 w551 w560 w639 w659 w693 w701 w715 w727 w733 _]
                    tunnel: w392 -> [_ w473 w483 w504 _ _ _ _ _ _ _ _ _ _ _ _]
                    tunnel: w405 -> [_ _ w494 _ w523 _ _ _ _ w676 _ w707 _ w728 _ _]
                    tunnel: w316 -> [_ _ w489 _ w508 w533 w547 w575 w642 w674 w690 w702 _ w725 _ _]
                    tunnel: [w459 w480 w498 w503 w527 w532 w552 w574 w646 w672 w694 w705 w715 w726 w733 states_def."tone after"] -> w308
                    tunnel: w391 -> [_ _ _ _ _ _ _ _ _ _ _ _ _ _ _ _]
                    tunnel: [w457 w475 w495 w499 w520 w531 w549 w566 w643 w664 w698 w699 w714 w719 w732 w736] -> w381
                    tunnel: w362 -> [_ _ _ _ _ _ _ w564 w647 w661 _ _ _ _ _ _]
                    tunnel: w331 -> [w453 w477 w497 w501 w526 w534 w550 w569 w645 w668 w691 w711 w716 w721 w735 w737]
                    tunnel: w390 -> [_ _ _ _ _ w536 _ _ _ _ _ _ _ _ _ _]
                    tunnel: w402 -> [w455 w478 w492 w502 w519 w537 w546 w570 w641 w666 w696 w710 w717 w724 w734 w738]
                    tunnel: [w455 w478 w485 w502 w509 w535 w548 w570 w640 w665 w687 w703 w717 w722 w734 w738] -> w401
                    tunnel: w389 -> [_ _ _ _ _ _ _ w572 _ _ _ _ _ _ _ _]
                    tunnel: w388 -> [_ _ _ _ _ _ _ w571 _ _ _ _ _ _ _ _]
                    tunnel: [w457 w475 w495 w499 w520 w530 w549 w566 w643 w670 w698 w699 w714 w719 w732 w736] -> w380
                    tunnel: [w457 w475 w495 w499 w520 w530 w549 w566 w643 w669 w698 w699 w714 w719 w732 w736] -> w378
                    tunnel: [w454 w477 w497 w501 w526 w534 w550 w569 w644 w668 w691 w711 w716 w721 w735 w737] -> w393
                    tunnel: w309 -> [_ _ _ _ w511 _ _ w568 _ _ _ _ _ _ _ _]
                    tunnel: w399 -> [_ _ _ _ _ _ _ w567 _ _ _ _ _ _ _ _]
                    tunnel: w315 -> [_ _ _ _ _ _ _ _ _ w667 _ _ _ _ _ _]
                    tunnel: w398 -> [_ _ _ _ _ _ _ _ _ _ _ _ _ w723 _ _]
                    tunnel: [w457 w475 w495 w499 w520 w530 w549 w566 w643 w664 w698 TRUE w714 w719 w732 w736] -> w312
                    tunnel: w394 -> [_ _ _ _ _ _ _ _ _ _ _ w700 _ _ _ _]
                    tunnel: w352 -> [_ _ _ _ w524 _ _ _ _ _ _ _ _ _ _ _]
                    tunnel: w350 -> [_ _ _ _ _ _ _ _ _ _ w688 _ _ _ _ _]
                    tunnel: w313 -> [_ _ _ _ _ _ _ w561 _ w658 _ _ _ _ _ w740]
                    tunnel: w304 -> [_ _ w490 _ _ _ _ _ _ _ _ _ _ _ _ _]
                    tunnel: w301 -> [_ _ _ _ w510 _ _ _ _ _ _ _ _ _ _ _]
                    frame 0, Default {
                      w457 = FALSE
                      n248 = local read "trialStart"() -> (w458:bool)
                      n249 = case shown="True" w458 {
                        tunnel: [w461 w464] -> w459
                        tunnel: w456 -> [w461 _]
                        tunnel: w453 -> [w460 w463]
                        tunnel: [w460 w462] -> w454
                        frame False {
                        }
                        frame True {
                          n250 = stacked-sequence {
                            tunnel: [w465 _] -> w464
                            tunnel: w463 -> [_ w471]
                            tunnel: [_ w470] -> w462
                            frame #0 {
                              n251 = local read "toneReward"() -> (w466:bool)
                              n252 = case shown="False" w466 {
                                tunnel: [states_def."tone" states_def."vs before"] -> w465
                                frame True {
                                }
                                frame False {
                                }
                              }
                            }
                            frame #1 {
                              w469 = FALSE
                              n253 = local write "trialStart"(w469) -> ()
                              n254 = local write "skipRewFlag"(w469) -> ()
                              n255 = Increment(x=w471) -> (x+1=w470:i32)
                            }
                          }
                        }
                      }
                    }
                    frame 1 {
                      w475 = FALSE
                      n256 = local read "No VS"() -> (w474:bool)
                      n257 = Or(x=w473, y=w474) -> (x .or. y?=w472:bool)
                      n258 = Select(t=states_def."vs", s=w472, f=w479) -> (s? t:f=w480:u32)
                    }
                    frame 2 {
                      w495 = FALSE
                      n259 = Not Equal?(x=w494, y=w493) -> (x != y?=w491:bool)
                      n260 = Select(t=w489, s=w491, f=w492) -> (s? t:f=w485:u64)
                      n261 = Add(x=w485, y=w490) -> (x+y=w488:u64)
                      n262 = local read "No VS"() -> (w481:bool)
                      n263 = Greater?(x=w489, y=w488) -> (0:w486:bool)
                      n264 = Or(x=w481, y=w486) -> (x .or. y?=w484:bool)
                      n265 = Not(x=w481) -> (.not. x?=w482:bool)
                      n266 = local write "actuatorOn"(w484) -> ()
                      n267 = And(x=w483, y=w482) -> (x .and. y?=w487:bool)
                      n268 = Select(t=w493, s=w487, f=states_def."delay") -> (s? t:f=w498:u32)
                    }
                    frame 3 {
                      w499 = FALSE
                      n269 = Select(t=w505, s=w504, f=states_def."delay") -> (s? t:f=w503:u32)
                    }
                    frame 4 {
                      w520 = FALSE
                      n270 = local read "allowPunish"() -> (w512:bool)
                      n271 = Not Equal?(x=w523, y=w522) -> (x != y?=w521:bool)
                      n272 = Select(t=w508, s=w521, f=w519) -> (s? t:f=w509:u64)
                      n273 = And(x=w512, y=w511) -> (x .and. y?=w513:bool)
                      n274 = case shown="True" w513 {
                        selector: w513 -> [_ w529]
                        frame False {
                        }
                        frame True {
                          n275 = local write "skipRewFlag"(w529) -> ()
                        }
                      }
                      n276 = Add(x=w524, y=w509) -> (x+y=w525:u64)
                      n277 = local read "skipRewFlag"() -> (w517:bool)
                      n278 = Less?(x=w525, y=w508) -> (x < y?=w518:bool)
                      n279 = Add(x=w509, y=w510) -> (x+y=w507:u64)
                      n280 = Select(t=states_def."timeout", s=w517, f=states_def."tone after") -> (s? t:f=w515:T5)
                      n281 = Greater?(x=w508, y=w507) -> (0:w506:bool)
                      n282 = case shown="True" w506 {
                        frame False {
                        }
                        frame True {
                          n283 = local write "actuatorOn"(TRUE) -> ()
                        }
                      }
                      n284 = Select(t=w515, s=w518, f=w522) -> (s? t:f=w527:u32)
                    }
                    frame 5 {
                      w530 = FALSE
                      n285 = case shown="True" w536 {
                        tunnel: [w539 states_def."tone after"] -> w532
                        tunnel: w538 -> [w539 _]
                        tunnel: w537 -> [w541 _]
                        tunnel: [w541 w544] -> w535
                        tunnel: w533 -> [_ w544]
                        tunnel: [TRUE FALSE] -> w531
                        frame False {
                        }
                        frame True {
                        }
                      }
                    }
                    frame 6 {
                      w549 = FALSE
                      n286 = local read "Busy"() -> (w545:bool)
                      n287 = case shown="True" w545 {
                        tunnel: [w554 states_def."tone after"] -> w552
                        tunnel: w551 -> [w554 _]
                        tunnel: w547 -> [_ w555]
                        tunnel: [w553 w555] -> w548
                        tunnel: w546 -> [w553 _]
                        frame False {
                        }
                        frame True {
                        }
                      }
                    }
                    frame 7 {
                      w566 = FALSE
                      n288 = local read "toneReward"() -> (w563:bool)
                      n289 = local read "allowAutoWater"() -> (w559:bool)
                      n290 = Or(x=w563, y=w564) -> (x .or. y?=w562:bool)
                      n291 = case shown="False" w568 {
                        tunnel: w572 -> [_ w600]
                        tunnel: w571 -> [_ w599]
                        tunnel: w562 -> [_ w598]
                        tunnel: w561 -> [_ w597]
                        tunnel: [w589 w595] -> w558
                        tunnel: w560 -> [w589 w593]
                        frame False {
                        }
                        frame True {
                          n292 = case shown="True" w598 {
                            tunnel: [w616 w630] -> w590
                            tunnel: w600 -> [w613 w629]
                            tunnel: w599 -> [w617 w628]
                            tunnel: w597 -> [_ w627]
                            frame True {
                              n293 = Not(x=w613) -> (.not. x?=w618:bool)
                              n294 = Not(x=w617) -> (.not. x?=w614:bool)
                              n295 = local read "rightcounter"() -> (w610:i32)
                              n296 = local read "leftcounter"() -> (w611:i32)
                              n297 = Select(t=3, s="forceLRswitch", f=inf) -> (s? t:f=w601:dbl)
                              n298 = Select(t=3, s="forceLRswitch", f=inf) -> (s? t:f=w607:dbl)
                              n299 = Less?(x=w610, y=w601) -> (x < y?=w609:bool)
                              n300 = Compound Arithmetic op=AND(w618, w617, w609) -> (w615:bool)
                              n301 = Less?(x=w611, y=w607) -> (x < y?=w612:bool)
                              n302 = Compound Arithmetic op=AND(w612, w613, w614) -> (w608:bool)
                              n303 = case shown="True" w608 {
                                frame False {
                                }
                                frame True {
                                n304 = local read "leftcounter"() -> (w624:i32)
                                n305 = local write "FlagWaterLeft"(TRUE) -> ()
                                n306 = Increment(x=w624) -> (x+1=w625:i32)
                                n307 = local write "leftcounter"(w625) -> ()
                                n308 = local write "rightcounter"(0) -> ()
                                }
                              }
                              n309 = case shown="True" w615 {
                                frame False {
                                }
                                frame True {
                                n310 = local read "rightcounter"() -> (w620:i32)
                                n311 = local write "FlagWaterLeft"(FALSE) -> ()
                                n312 = Increment(x=w620) -> (x+1=w619:i32)
                                n313 = local write "rightcounter"(w619) -> ()
                                n314 = local write "leftcounter"(0) -> ()
                                }
                              }
                              n315 = Exclusive Or(1:w615, 2:w608) -> (0:w616:bool)
                            }
                            frame False {
                              # "Consider add another state for automaticaly give water \nwhen animal did not get water for consecutively 10 trials?"
                              n316 = case shown="2" w627 {
                                tunnel: [w633 w635] -> w630
                                tunnel: w629 -> [w632 w638]
                                tunnel: w628 -> [w631 w636]
                                frame 1, Default {
                                # "left"
                                n317 = Not(x=w631) -> (.not. x?=w634:bool)
                                n318 = And(x=w632, y=w634) -> (x .and. y?=w633:bool)
                                }
                                frame 2 {
                                # "right"
                                n319 = Not(x=w638) -> (.not. x?=w637:bool)
                                n320 = And(x=w637, y=w636) -> (x .and. y?=w635:bool)
                                }
                              }
                            }
                          }
                          n321 = local read "allowCorrection"() -> (w592:bool)
                          n322 = Select(t=w593, s=w592, f=states_def."timeout") -> (s? t:f=w591:u32)
                          n323 = Select(t=states_def."reward", s=w590, f=w591) -> (s? t:f=w595:u32)
                        }
                      }
                      n324 = case shown="True" w559 {
                        tunnel: w558 -> [w577 w587]
                        tunnel: [w577 w586] -> w557
                        frame False {
                        }
                        frame True {
                          w580 = 10 ("Priority")
                          n325 = local read "contNoReward"() -> (w584:i32)
                          n326 = Random Number (0-1)() -> (number: 0 to 1=w581:dbl)
                          n327 = Multiply(x=w581, y=w580) -> (x*y=w579:dbl)
                          n328 = Add(x=w579, y=w580) -> (x+y=w578:dbl)
                          n329 = Greater Or Equal?(x=w584, y=w578) -> (x >= y?=w583:bool)
                          n330 = Select(t=0 ("Priority"), s=w583, f=w584) -> (s? t:f=w582:i32)
                          n331 = Select(t=states_def."manualwater", s=w583, f=w587) -> (s? t:f=w586:u32)
                          n332 = local write "contNoReward"(w582) -> ()
                        }
                      }
                      n333 = Add(x=w567, y=w570) -> (x+y=w576:u64)
                      n334 = Greater?(x=w575, y=w576) -> (0:w573:bool)
                      n335 = Select(t=states_def."cycle end", s=w573, f=w557) -> (s? t:f=w574:u32)
                    }
                    frame 8 {
                      w643 = FALSE
                      # "inform host computer to start \nanother trial"
                      n336 = case shown="True" w647 {
                        tunnel: [w649 w655] -> w644
                        tunnel: [states_def."idle" states_def."tone after"] -> w646
                        tunnel: w645 -> [w649 w655]
                        tunnel: [w650 w653] -> w640
                        tunnel: w642 -> [w650 w653]
                        tunnel: w641 -> [_ _]
                        tunnel: w639 -> [_ _]
                        frame False {
                          n337 = local write "actuatorOn"(FALSE) -> ()
                          n338 = local write "trialDone"(TRUE) -> ()
                        }
                        frame True {
                        }
                      }
                    }
                    frame 9 {
                      w664 = FALSE
                      w656 = states_def."reward refractory"
                      n339 = Not Equal?(x=w676, y=w659) -> (x != y?=w671:bool)
                      n340 = local read "toneReward"() -> (w662:bool)
                      n341 = Select(t=w674, s=w671, f=w666) -> (s? t:f=w665:u64)
                      n342 = Or(x=w661, y=w662) -> (x .or. y?=w663:bool)
                      n343 = case shown="False" w663 {
                        tunnel: [w678 w681] -> w670
                        tunnel: [w677 w680] -> w669
                        tunnel: w658 -> [_ w679]
                        frame True {
                          n344 = local read "FlagWaterLeft"() -> (w678:bool)
                          n345 = Not(x=w678) -> (.not. x?=w677:bool)
                        }
                        frame False {
                          n346 = case shown="0, Default" w679 {
                            tunnel: [w682 w684 w685] -> w681
                            tunnel: [w682 w683 w686] -> w680
                            frame 0, Default {
                              w682 = FALSE
                            }
                            frame 1 {
                              w684 = TRUE
                              n347 = Not(x=w684) -> (.not. x?=w683:bool)
                            }
                            frame 2 {
                              w686 = TRUE
                              n348 = Not(x=w686) -> (.not. x?=w685:bool)
                            }
                          }
                        }
                      }
                      n349 = Add(x=w667, y=w665) -> (x+y=w675:u64)
                      n350 = Less?(x=w675, y=w674) -> (x < y?=w673:bool)
                      n351 = Select(t=w656, s=w661, f=states_def."cycle end") -> ()  [unwired: 1 out]
                      n352 = local write "rewardStatus"(TRUE) -> ()
                      n353 = Select(t=w656, s=w673, f=w659) -> (s? t:f=w672:u32)
                    }
                    frame 10 {
                      w698 = FALSE
                      n354 = Not Equal?(x=w693, y=w693) -> (x != y?=w697:bool)
                      n355 = Select(t=w690, s=w697, f=w696) -> (s? t:f=w687:u64)
                      n356 = Add(x=w687, y=w688) -> (x+y=w689:u64)
                      n357 = Greater?(x=w690, y=w689) -> (0:w695:bool)
                      n358 = Select(t=states_def."cycle end", s=w695, f=w693) -> (s? t:f=w694:u32)
                    }
                    frame 11 {
                      w699 = FALSE
                      n359 = Not Equal?(x=w707, y=w701) -> (x != y?=w709:bool)
                      n360 = case shown="True" w709 {
                        tunnel: w701 -> [_ w713]
                        frame False {
                        }
                        frame True {
                          "curState" <- w713
                        }
                      }
                      n361 = Select(t=w702, s=w709, f=w710) -> (s? t:f=w703:u64)
                      n362 = Add(x=w703, y=w700) -> (x+y=w704:u64)
                      n363 = Less?(x=w702, y=w704) -> (x < y?=w708:bool)
                      n364 = local read "curState"() -> (w706:u32)
                      n365 = Select(t=w701, s=w708, f=w706) -> (s? t:f=w705:u32)
                    }
                    frame 12 {
                      w714 = FALSE
                      # "To do"
                    }
                    frame 13 {
                      w719 = FALSE
                      # "To do: change the state when timeout finished?????"
                      n366 = Not Equal?(x=w728, y=w727) -> (x != y?=w731:bool)
                      n367 = Select(t=w725, s=w731, f=w724) -> (s? t:f=w722:u64)
                      n368 = local write "actuatorOn"(FALSE) -> ()
                      n369 = Add(x=w722, y=w723) -> (x+y=w730:u64)
                      n370 = Greater?(x=w725, y=w730) -> (0:w729:bool)
                      n371 = Select(t=states_def."cycle end", s=w729, f=w727) -> (s? t:f=w726:u32)
                    }
                    frame 14 {
                      w732 = FALSE
                    }
                    frame 15 {
                      w736 = FALSE
                      n372 = case shown="1" w740 {
                        frame 0, Default {
                        }
                        frame 1 {
                          n373 = local write "manualWaterLeft"(TRUE) -> ()
                        }
                        frame 2 {
                          n374 = local write "manualWaterRight"(TRUE) -> ()
                        }
                      }
                    }
                  }
                  n375 = local read "rtFIFOdataPool"() -> (w358:u32)
                  n376 = local read "rtFIFOdataDim"() -> (w363:i32)
                  n377 = Multiply(x=w363, y=w358) -> (x*y=w364:u32)
                  n378 = local read "manualWaterRight"() -> (w319:bool)
                  n379 = case shown="False" w319 {
                    tunnel: [w416 w425] -> w317
                    tunnel: w318 -> [w417 _]
                    tunnel: w316 -> [w415 w425]
                    tunnel: w315 -> [w414 _]
                    frame False {
                      n380 = local read "rightWaterOnFlag"() -> (w413:bool)
                      n381 = case shown="True" w413 {
                        tunnel: w417 -> [_ w422]
                        tunnel: [0 w422] -> w416
                        tunnel: w415 -> [_ w424]
                        tunnel: w414 -> [_ w423]
                        frame False {
                        }
                        frame True {
                          n382 = Add(x=w423, y=w422) -> (x+y=w421:u64)
                          n383 = Greater?(x=w424, y=w421) -> (0:w420:bool)
                          n384 = Not(x=w420) -> (.not. x?=w419:bool)
                          n385 = local write "rightWaterOnFlag"(w419) -> ()
                        }
                      }
                    }
                    frame True {
                      n386 = local write "manualWaterRight"(FALSE) -> ()
                      n387 = local write "rightWaterOnFlag"(TRUE) -> ()
                    }
                  }
                  n388 = shared-variable ".\\variables - network - RT (separate).lvlib\\stop - network"() -> (w410:bool)  [unwired: 1 in, 1 out]
                  n389 = local read "leftWaterOnFlag"() -> (w320:bool)
                  n390 = local read "rightWaterOnFlag"() -> (w314:bool)
                  n391 = local read "allowPunish"() -> (w310:bool)
                  n392 = local read "actuatorOn"() -> (w311:bool)
                  n393 = Select(t=states_def."exit", s=w410, f=w308) -> (s? t:f=w400:u32)
                  n394 = feedback-in #2(w400) -> ()
                  n395 = feedback-in #3(w400) -> ()
                  n396 = call "punish_check.vi"("input state"=w308, "lick"=w309, "allow punish"=w310) -> ("punish"=w307:bool)
                  n397 = Or(x=w320, y=w380) -> (x .or. y?=w379:bool)
                  n398 = Or(x=w314, y=w378) -> (x .or. y?=w377:bool)
                  n399 = Compound Arithmetic op=OR(w307, w311, w312) -> (w397:bool)
                  n400 = local read "ABORT"() -> (w344:bool)
                  n401 = Build Array(w381, w379, w377, w397) -> (w373:bool[])
                  n402 = Build Array (concatenate)(w376, w373, w375) -> (w374:bool[])
                  n403 = Boolean Array To Number(Boolean array=w374) -> (number=w326:u32)
                  n404 = Build Array (concatenate)(w367, w326, w324) -> (w365:dbl[])
                  n405 = Array Size(array=w365) -> (size(s)=w346:i32)
                  n406 = Build Array (concatenate)(w387, w365) -> (w385:dbl[])
                  n407 = local write "rtFIFOdataDim"(w346) -> ()
                  n408 = Array Size(array=w385) -> (size(s)=w382:i32)
                  n409 = Equal?(x=w382, y=w364) -> (x = y?=w384:bool)
                  n410 = Not Equal?(x=w346, y=9) -> (x != y?=w345:bool)
                  n411 = case shown="False" w384 {
                    tunnel: [w445 w452] -> w383
                    tunnel: w385 -> [w446 w449]
                    tunnel: [w446 sgl[] [] ("array type (2D Dbl)")] -> w386
                    tunnel: w360 -> [_ w448]
                    tunnel: w359 -> [w445 w447]
                    frame False {
                    }
                    frame True {
                      n412 = local read "rtFIFOtimeout"() -> (w450:u32)
                      n413 = RT FIFO Write(0:w448, 1:w449, 2:w450, 3:w447) -> (11:w452:errorcluster)  [unwired: 1 in, 3 out]
                    }
                  }
                  n414 = case shown="False" w345 {
                    frame False {
                    }
                    frame True {
                      n415 = One Button Dialog(message="The dimention of rtFIFOdata is not 4, pleae change the size of alocated network stream.") -> (true=w443:bool)  [unwired: 1 in]
                      n416 = local write "ABORT"(w443) -> ()
                    }
                  }
                  n417 = call-poly <vilib>:"DAQmx Write.vi"("task/channels in"=w349, "data"=w373, "error in"=w348) -> ("task out"=w404:refnum<k21>, "error out"=w403:errorcluster)  [unwired: 10 in, 1 out]
                  n418 = node-c288() -> ()  [unwired: 1 in, 1 out]
                }
                n419 = node-c288(5.0, 100 ("Priority")) -> (w232:T2)  [unwired: 1 in]
                n420 = timed-loop {
                  timing: w232 -> [_]
                  timing-out: [_] -> w231
                  tunnel: [w272] -> w209
                  tunnel: [w271] -> w208
                  tunnel: [w270] -> w211
                  tunnel: [w269] -> w210
                  tunnel: w230 -> [w268]
                  tunnel: w229 -> [w267]
                  tunnel: w216 -> [w266]
                  tunnel: w215 -> [w265]
                  shift-right: [w275] -> _
                  shift-left: w225 -> [w274]
                  stop <- w273 stop-if-true
                  n421 = node-c288() -> ()  [unwired: 1 in, 1 out]
                  n422 = property class="Network Stream Endpoint"(reference=w267, error in=w268) -> (reference out=w277:refnum<k21>, error out=w276:errorcluster, "Connected"=→"Is Connected":bool, "AvailElmntsForWrite"=→"Available Elements for Writing":i32)
                  n423 = RT FIFO Read(0:w266, 2:0, 3:w265) -> (8:w270:refnum<k33>, 9:w263:sgl[], 11:w269:errorcluster)  [unwired: 1 in, 2 out]
                  n424 = Empty Array?(array=w263) -> (empty?=w262:bool)
                  n425 = case shown="True" w262 {
                    tunnel: w263 -> [w285 _]
                    tunnel: [FALSE w290] -> w273
                    tunnel: w277 -> [w287 w288]
                    tunnel: w276 -> [w286 w289]
                    tunnel: [w280 w291] -> w275
                    tunnel: w274 -> [w283 w291]
                    tunnel: [w282 w288] -> w272
                    tunnel: [w281 w289] -> w271
                    frame False {
                      n426 = Increment(x=w283) -> (x+1=w280:i32)
                      n427 = shared-variable-write(w287, w286, w285) -> (w282:refnum<k21>, w281:errorcluster)  [unwired: 1 in, 1 out]
                      n428 = local write "stream counter"(w280) -> ()
                    }
                    frame True {
                      n429 = local read "ABORT"() -> (w290:bool)
                    }
                  }
                  n430 = node-c288() -> ()  [unwired: 1 in, 1 out]
                }
                n431 = node-c288(w231) -> (w199:errorcluster)
                n432 = node-c288(w235) -> (w201:errorcluster)
                n433 = Flush Stream(8:w208, 11:w209) -> (0:w207:errorcluster, 3:w206:refnum<k21>)  [unwired: 2 in, 1 out]
                n434 = RT FIFO Delete(0:w211, 3:w210) -> (11:w204:errorcluster)  [unwired: 1 in]
                n435 = Destroy Stream Endpoint(8:w207, 11:w206) -> (0:w205:errorcluster)
                n436 = node-c288(w233) -> (w200:errorcluster)
                n437 = stacked-sequence {
                  tunnel: w205 -> [w243]
                  tunnel: [w243] -> w198
                  frame #0 {
                    n438 = shared-variable "Sabrina-RT1\\variables - network - RT (separate).lvlib\\stop - network"(TRUE ("stop - network")) -> ()  [unwired: 1 in, 1 out]
                  }
                }
                n439 = Build Array(w196, w196, w196, w196) -> (w195:bool[])
                n440 = call-poly <vilib>:"DAQmx Write.vi"("task/channels in"=w203, "data"=w195, "error in"=w202) -> ("task out"=w176:refnum<k21>, "error out"=w175:errorcluster)  [unwired: 10 in, 1 out]
                n441 = call <vilib>:"DAQmx Stop Task.vi"("task/channels in"=w178, "error in"=w177) -> ("error out"=w174:errorcluster)  [unwired: 12 in, 1 out]
                n442 = call <vilib>:"DAQmx Stop Task.vi"("task/channels in"=w176, "error in"=w175) -> ("error out"=w173:errorcluster)  [unwired: 12 in, 1 out]
                n443 = Merge Errors(w193, w204) -> (w197:errorcluster)
                n444 = Merge Errors(w174, w173) -> (w179:errorcluster)
                n445 = Merge Errors(w201, w200, w199) -> (w180:errorcluster)
                n446 = Merge Errors(w180, w179, w197, w198) -> (w194:errorcluster)
                "error out" <- w194
                n447 = call <vilib>:"Simple Error Handler.vi"("error in (no error)"=w194) -> ()  [unwired: 4 in, 5 out]
              }
            }
          }
          frame #2 {
            n448 = Wait (ms)(milliseconds to wait=u32 100) -> ()  [unwired: 1 out]
          }
        }
      }
      n449 = UDP Close(connection ID=w24, 8:w23) -> (error out=w25:errorcluster)  [unwired: 1 out]
      n450 = UDP Close(connection ID=w19, 8:w20) -> (error out=w18:errorcluster)  [unwired: 1 out]
      n451 = call <vilib>:"Simple Error Handler.vi"("error in (no error)"=w25) -> ()  [unwired: 4 in, 5 out]
      n452 = call <vilib>:"Simple Error Handler.vi"("error in (no error)"=w18) -> ()  [unwired: 4 in, 5 out]
    }
  }
